vi "Close.vi"(8 "error in (no error)":errorcluster, 11 "reference in":refnum<class "LCR_BK891.lvclass">) -> (0 "error out":errorcluster, 3 "reference in":refnum<class "LCR_BK891.lvclass">)   [LabVIEW 2022 SP3, in "LCR_BK891.lvlib" / "LCR_BK891.lvclass"]
uses:
  LCR_BK891.lvclass
  Components/ViPER.lvlibp/ViPER.lvclass
  C:/Projects/Medulla/ViPER/Examples/Flux_Capacitor_Tester/Components/ViPER.lvlibp/ViPER.lvclass
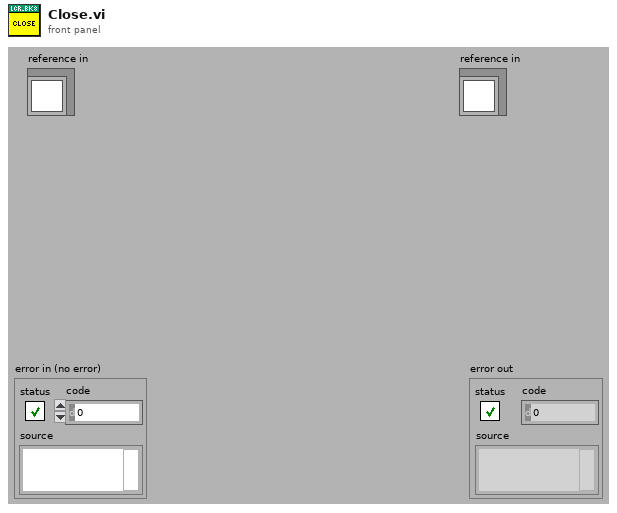
[diagram p1: front panel]
types:
  T1 = typedef "LCR_BK891.lvlib/LCR_BK891.lvclass/ObjectAttributes.ctl" = cluster{"Config":T2, "VISA Ref":refnum<visa-resource-name>, "Function":u16, "Range":u16, "Measurement Speed":u16, "Signal Frequency":dbl, "Signal Level":u8, "Measured Primary Reading":dbl, "Measured Secondary Reading":dbl}
  T2 = typedef "LCR_BK891.lvlib/LCR_BK891.lvclass/Config.ctl" = cluster{"VISA":refnum<visa-resource-name>}
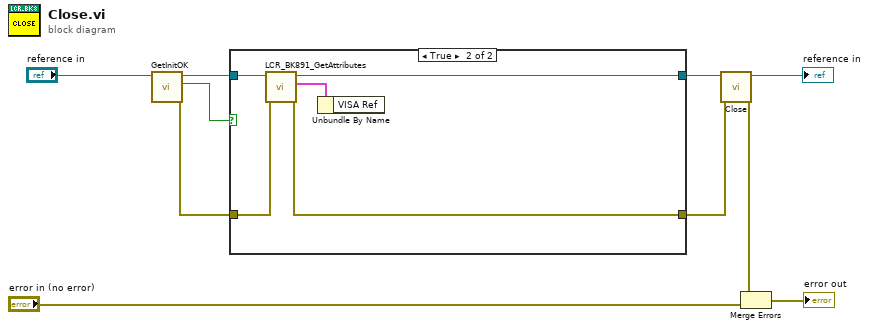
[diagram p0: block diagram]
diagram:
  n1 = call "GetInitOK.vi"("reference in"="reference in") -> ("error out"=w4:errorcluster, "init_ok"=w5:bool, "reference out"=w6:refnum<class "LCR_BK891.lvclass">)  [unwired: 8 in]
  n2 = case shown="True" w5 {
    tunnel: w4 -> [w12 w16]
    tunnel: [w12 w13] -> w7
    tunnel: w6 -> [w11 w17]
    tunnel: [w11 w14] -> w8
    frame False {
    }
    frame True {
      n3 = call "LCR_BK891_GetAttributes.vi"("error in (no error)"=w16, "reference in"=w17) -> ("error out"=w13:errorcluster, "Data"=w15:T1, "reference out"=w14:refnum<class "LCR_BK891.lvclass">)  [unwired: 6 in, 1 out]
      n4 = Unbundle By Name(w15) -> ()  [unwired: 1 out]
    }
  }
  n5 = call-parent "Close.vi"("error in (no error)"=w7, "reference in"=w8) -> ("error out"=w3:errorcluster, "reference out"=→"reference in":refnum<class "LCR_BK891.lvclass">)  [unwired: 8 in]
  n6 = Merge Errors(w3, "error in (no error)") -> (→"error out":errorcluster)
